vi "Base10 To Base32.vi"(2 "Base 10":u64) -> (0 "Base32":string, 1 "length":i32)   [LabVIEW 2016]
panel:
  out "Array":u8[](array[numeric])
  out "size(s)":i32
  out "Base 10":u64 format="%#_16f"
  # "No 1, I, 0 or O"
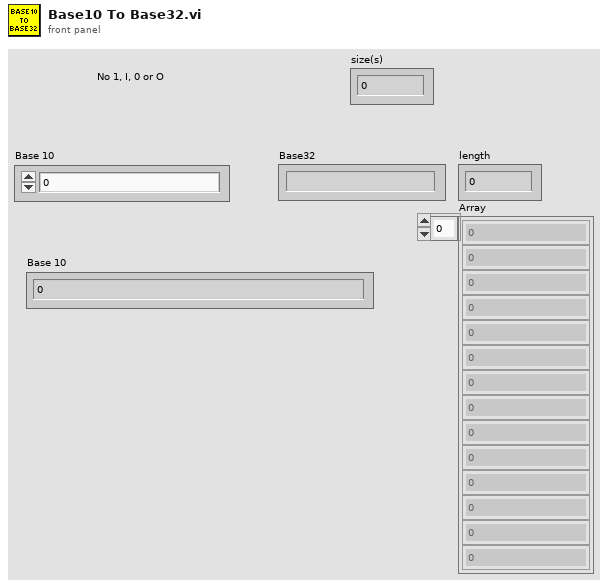
[diagram p1: front panel]
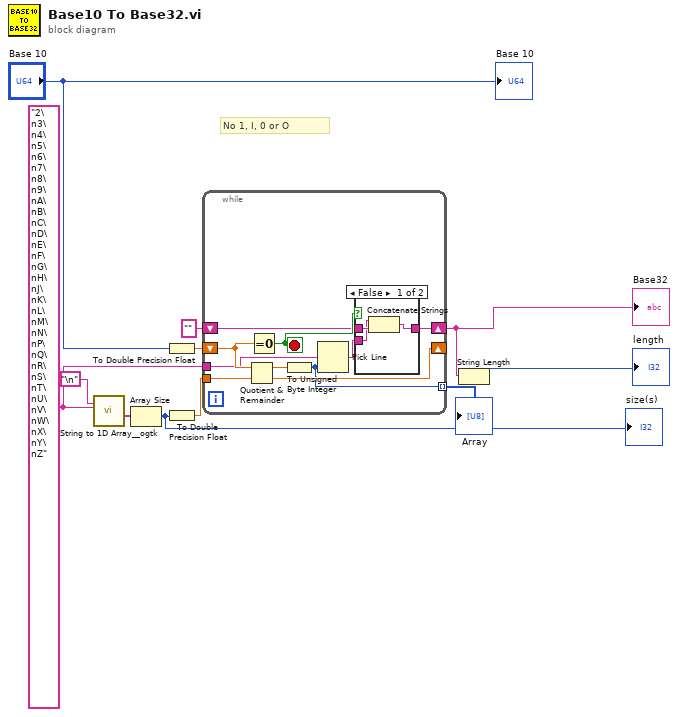
[diagram p0: block diagram]
diagram:
  w8 = "2\n3\n4\n5\n6\n7\n8\n9\nA\nB\nC\nD\nE\nF\nG\nH\nJ\nK\nL\nM\nN\nP\nQ\nR\nS\nT\nU\nV\nW\nX\nY\nZ" ("multi-line string")
  # "No 1, I, 0 or O"
  n1 = call <userlib>:"String to 1D Array__ogtk.vi"("delimiter (Tab)"="\n", "string"=w8) -> ("Array of Strings"=w7:string[])  [unwired: 9 in]
  n2 = Array Size(array=w7) -> (size(s)=w5:i32)
  "size(s)" <- w5
  n3 = To Double Precision Float(number="Base 10") -> (double precision float=w10:dbl)
  n4 = To Double Precision Float(number=w5) -> (double precision float=w4:dbl)
  n5 = while {
    shift-right: [w19] -> _
    shift-left: w10 -> [w21]
    tunnel: w8 -> [w17]
    tunnel: w4 -> [w16]
    shift-right: [w15] -> w2
    shift-left: "" -> [w14]
    tunnel: [w12] -> w1 mode=indexing
    stop <- w18 stop-if-true
    n6 = Quotient & Remainder(x=w21, y=w16) -> (x-y*floor(x/y)=w20:dbl, floor(x/y)=w19:dbl)
    n7 = Equal To 0?(x=w21) -> (x = 0?=w18:bool)
    n8 = To Unsigned Byte Integer(number=w20) -> (unsigned 8bit integer=w12:u8)
    n9 = Pick Line(multi-line string=w17, line index=w12) -> (output string=w13:string)  [unwired: 1 in]
    n10 = case shown="False" w18 {
      tunnel: [w23 w25] -> w15
      tunnel: w14 -> [w24 w25]
      tunnel: w13 -> [w22 _]
      frame False {
        n11 = Concatenate Strings(w22, w24) -> (w23:string)
      }
      frame True {
      }
    }
  }
  "Base32" <- w2
  "Array" <- w1
  n12 = String Length(string=w2) -> (length=→"length":i32)
  "Base 10" <- "Base 10"
